vi "HTTP Method_core.vi"(0 "REST Client_NET in":refnum<class "REST Client_NET.lvclass">, 1 "Method":T2, 5 "Resolved URL":string, 7 "Request body":string, 9 "Multipart Post data":T1[](array[typedef]), 11 "error in (no error)":errorcluster, 12 "request specific headers":T3[](array[typedef]), 13 "timeout (0 = Use Default)":i32) -> (2 "ReasonPhrase":string, 3 "StatusCode":i32, 4 "REST Client_NET out":refnum<class "REST Client_NET.lvclass">, 6 "REST Client Headers_NET out":refnum<class "REST Client Headers_NET.lvclass">, 8 "Response":string, 15 "error out":errorcluster)   [LabVIEW 2018, in "REST Client_NET.lvlib" / "REST Client_NET.lvclass"]
doc: "<b> </b> <b> </b>\nHttpClient_NET\nJustin Young - Viviota\nCopyright (c) 2021\nLicense: BSD"
uses:
  REST Client_NET.lvclass
  Rest Client Headers_NET/REST Client Headers_NET.lvclass
  <vilib>/addons/_JKI.lib/REST Client/classes/REST Client/HTTP Header.ctl
  <vilib>/addons/_JKI.lib/REST Client/classes/REST Client/HTTP Methods.ctl
  <vilib>/httpClient/MultipartData.ctl
  Types/HttpNet_error_enum.ctl
  REST Client_NET.lvclass/REST Client_NET.ctl
  HttpHeaders_response/HttpHeaders_Response.lvclass
  HttpHeaders_content/HttpHeaders_Content.lvclass
  LabVIEWHTTPClient_NET/HttpClient_NET.lvclass
  HttpClient_NET.lvlib
  <vilib>/addons/_JKI.lib/REST Client/classes/REST Client/REST Client.lvclass
  <vilib>/httpClient/LabVIEWHTTPClient.lvlib
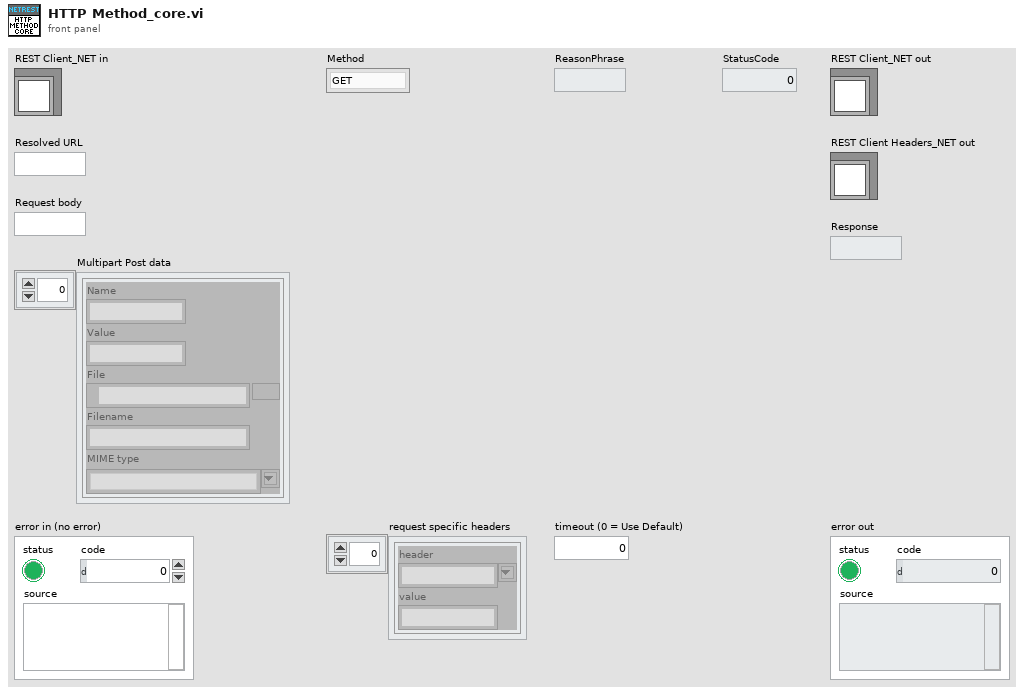
[diagram p1: front panel]
types:
  T1 = typedef "LabVIEWHTTPClient.lvlib/MultipartData.ctl" = cluster{"Name":string, "Value":string, "File":path, "Filename":string, "MIME type":string}
  T2 = typedef "REST Client.lvlib/REST Client.lvclass/HTTP Methods.ctl" = enum16{"GET", "HEAD", "POST", "PUT", "DELETE"}
  T3 = typedef "REST Client.lvlib/REST Client.lvclass/HTTP Header.ctl" = cluster{"header":string, "value":string}
  T4 = typedef "HttpClient_NET.lvlib/HttpNet_error_enum.ctl" = enum16{"REST method is not available", "URL cannot be blank", "Output filepath cannot be empty", "Input filepath cannot be empty", "Internal .NET error %s", "Output filepath cannot be directory", "Download Task no longer exists", "Mutipart Put not supported from REST Client Interface.  Please revert to lower level classes"}
  T5 = typedef "HttpClient_NET.lvlib/method_enum.ctl" = enum16{"GET", "PUT", "POST", "DELETE", "HEAD", "TRACE", "SEND"}
  T6 = typedef "HttpClient_NET.lvlib/ResponseHeaders_Cluster.ctl" = cluster{"ResponseHeader":refnum<class "HttpHeaders_Response.lvclass">, "ContentHeaders":refnum<class "HttpHeaders_Content.lvclass">}
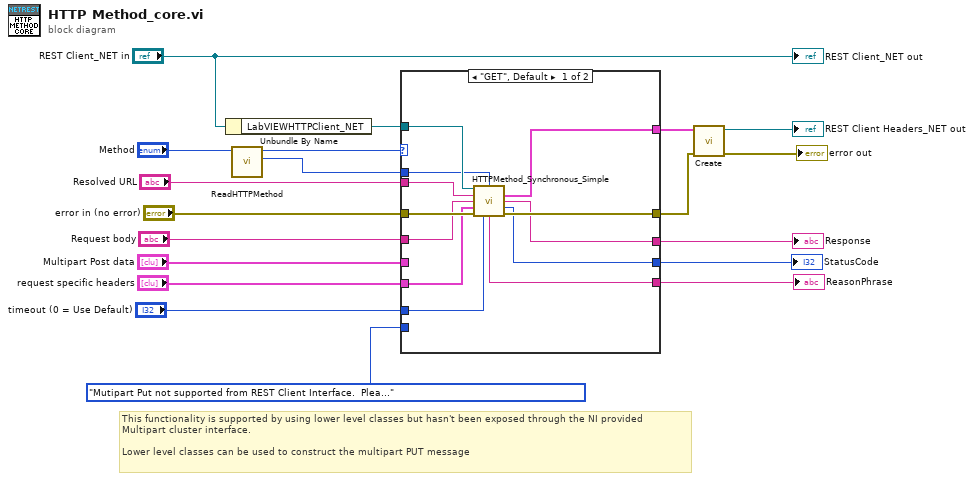
[diagram p0: block diagram]
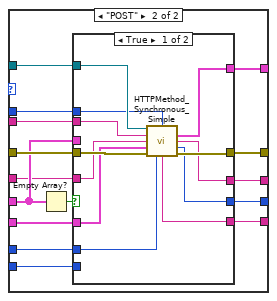
[diagram p2: hidden frame]
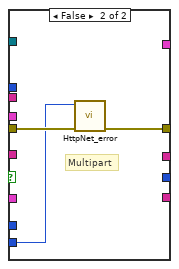
[diagram p3: hidden frame]
diagram:
  # "This functionality is supported by using lower level classes but hasn't been exposed through the NI provided\nMultipart cluster interface. \n\nLower level classes can be used to construct the multipart PUT message"
  n1 = Unbundle By Name("REST Client_NET in") -> ("LabVIEWHTTPClient_NET"=w14:refnum<class "HttpClient_NET.lvclass">)
  n2 = call "ReadHTTPMethod.vi"("Method"="Method") -> ("HTTP method_NET"=w1:T5, "HTTP method"=w2:T2)  [unwired: 9 in]
  n3 = case shown="\"GET\", Default" w2 {
    tunnel: [w25 w46] -> w18
    tunnel: "Resolved URL" -> [w28 w45]
    tunnel: [w27 w44] -> w11
    tunnel: [w29 w43] -> w5
    tunnel: "timeout (0 = Use Default)" -> [w21 w42]
    tunnel: "error in (no error)" -> [w30 w40]
    tunnel: w14 -> [w31 w39]
    tunnel: [w26 w34] -> w15
    tunnel: "request specific headers" -> [w24 w38]
    tunnel: [w23 w35] -> w17
    tunnel: "Multipart Post data" -> [_ w37]
    tunnel: "Request body" -> [w22 w36]
    tunnel: HttpNet_error_enum."Mutipart Put not supported from REST Client Interface.  Please revert to lower level classes" ("Error") -> [_ w33]
    tunnel: w1 -> [w20 w32]
    frame "GET", Default {
      n4 = call "HTTPMethod_Synchronous_Simple.vi"("LabVIEWHTTPClient_NET in"=w31, "Method"=w20, "URL"=w28, "buffer"=w22, "request headers"=w24, "error in (no error)"=w30, "Timeout_ms (10000)"=w21) -> ("Headers"=w25:T6, "Response"=w27:string, "StatusCode"=w26:i32, "ReasonPhrase"=w23:string, "error out"=w29:errorcluster)  [unwired: 2 in, 2 out]
    }
    frame "POST" {
      n5 = Empty Array?(array=w37) -> (empty?=w41:bool)
      n6 = case shown="True" w41 {
        tunnel: w45 -> [w56 _]
        tunnel: w42 -> [w52 _]
        tunnel: w40 -> [w58 w61]
        tunnel: [w54 _] -> w46
        tunnel: [w53 _] -> w44
        tunnel: [w57 w60] -> w43
        tunnel: w37 -> [_ _]
        tunnel: w39 -> [w55 _]
        tunnel: w38 -> [w51 _]
        tunnel: w36 -> [w50 _]
        tunnel: [w49 _] -> w35
        tunnel: [w48 _] -> w34
        tunnel: w33 -> [_ w59]
        tunnel: w32 -> [w47 _]
        frame True {
          n7 = call "HTTPMethod_Synchronous_Simple.vi"("LabVIEWHTTPClient_NET in"=w55, "Method"=w47, "URL"=w56, "buffer"=w50, "request headers"=w51, "error in (no error)"=w58, "Timeout_ms (10000)"=w52) -> ("Headers"=w54:T6, "Response"=w53:string, "StatusCode"=w48:i32, "ReasonPhrase"=w49:string, "error out"=w57:errorcluster)  [unwired: 2 in, 2 out]
        }
        frame False {
          # "Multipart"
          n8 = call "HttpNet_error.vi"("Error In"=w61, "Error"=w59) -> ("Error Out"=w60:errorcluster)  [unwired: 9 in]
        }
      }
    }
  }
  "ReasonPhrase" <- w17
  "StatusCode" <- w15
  "Response" <- w11
  n9 = call "Create.vi"("error in (no error)"=w5, "Headers"=w18) -> ("error out"=→"error out":errorcluster, "REST Client Headers_NET out"=→"REST Client Headers_NET out":refnum<class "REST Client Headers_NET.lvclass">)  [unwired: 8 in]
  "REST Client_NET out" <- "REST Client_NET in"
